vi "sedSpectrometer_getSample_SaturationIsTrue.vi"(8 "error in (no error)":errorcluster, 11 "SaturationIsTrue_Ctl":T1) -> (0 "error out":errorcluster, 2 "function return":i32, 3 "SaturationIsTrue_Ctl out":T1)   [LabVIEW 2016, in "SALLV_sedSpectrometer.lvlib"]
doc: "int sedSpectrometer_shm_getSample_SaturationIsTrueLV(sedSpectrometer_SaturationIsTrueLV *SaturationIsTrue_Ctl );"
uses:
  SALLV_sedSpectrometer.lvlib
  DataTypes/SaturationIsTrue.ctl
  SALLV_sedSpectrometer.so
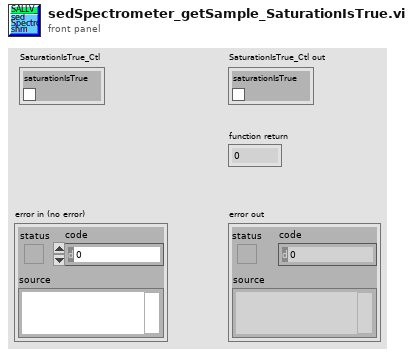
[diagram p1: front panel]
types:
  T1 = typedef "SALLV_sedSpectrometer.lvlib/SaturationIsTrue.ctl" = cluster{"saturationIsTrue":bool}
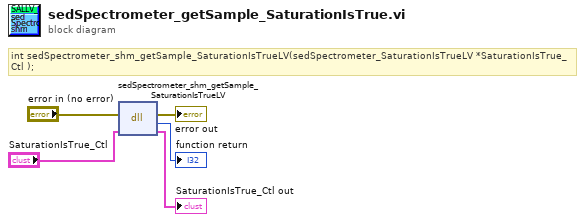
[diagram p0: block diagram]
diagram:
  # "int sedSpectrometer_shm_getSample_SaturationIsTrueLV(sedSpectrometer_SaturationIsTrueLV *SaturationIsTrue_Ctl );"
  n1 = dll-call lib="home/harini/TCS/SALLV_sedSpectrometer/SALLV_sedSpectrometer.*" fn="sedSpectrometer_shm_getSample_SaturationIsTrueLV"(error in="error in (no error)", "SaturationIsTrue_Ctl"="SaturationIsTrue_Ctl") -> (error out=→"error out":errorcluster, →"function return":i32, "SaturationIsTrue_Ctl"=→"SaturationIsTrue_Ctl out":T1)  [unwired: 2 in, 1 out]
